vi "Main_FPGA_r1.vi"() -> ()   [LabVIEW 2018]
uses:
  <vilib>/rvi/Emulation/niFpgaGetClockAttributes.vi
  <vilib>/rvi/Emulation/niFpgaSctlEmulationGetInTimedLoop.vi
  <vilib>/rvi/Emulation/niFpgaEmulationReportErrorSimple.vi
  <vilib>/rvi/Emulation/niFpgaCriticalErrorInLSC.vi
  <vilib>/rvi/Emulation/niFpgaProcessEmulError.vi
  SubVI/24AIO/AO/AO_FPGA.lvlib
  SubVI/24AIO/AI/AI_FPGA.lvlib
panel:
  out "AI19-26[]":i16[](array[numeric])
  out "AI10-17[]":i16[](array[numeric])
  out "AI1-8[]":i16[](array[numeric])
  in  "InitializeAI?":bool caption="Initialize?"
  in  "AO_Data(U32)":u32
  # "AI"
  # "AO"
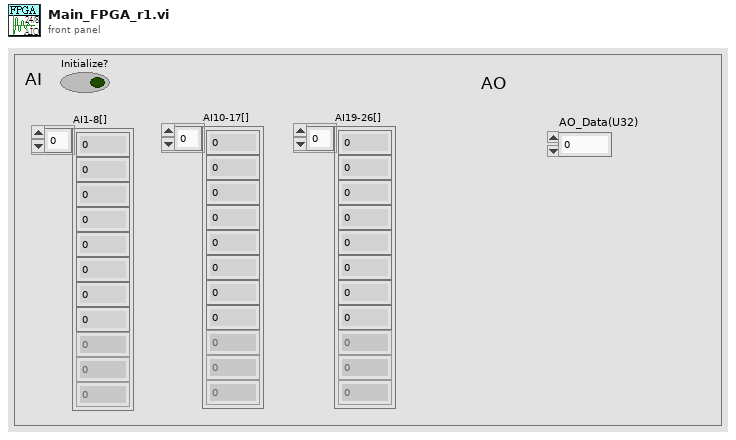
[diagram p1: front panel]
types:
  T1 = cluster{"CS":refnum<k21>, "CLK":refnum<k21>, "MOSI":refnum<k21>}
  T2 = cluster{"CONV":refnum<k21>, "RST":refnum<k21>, "SCK":refnum<k21>, "CS":refnum<k21>, "BUSY":refnum<k21>, "DOUT_A":refnum<k21>, "DOUT_B":refnum<k21>, "t_RST (ticks)":u32, "t_CONV (ticks)":u32, "t_BUSYMAX (ticks)":u32}
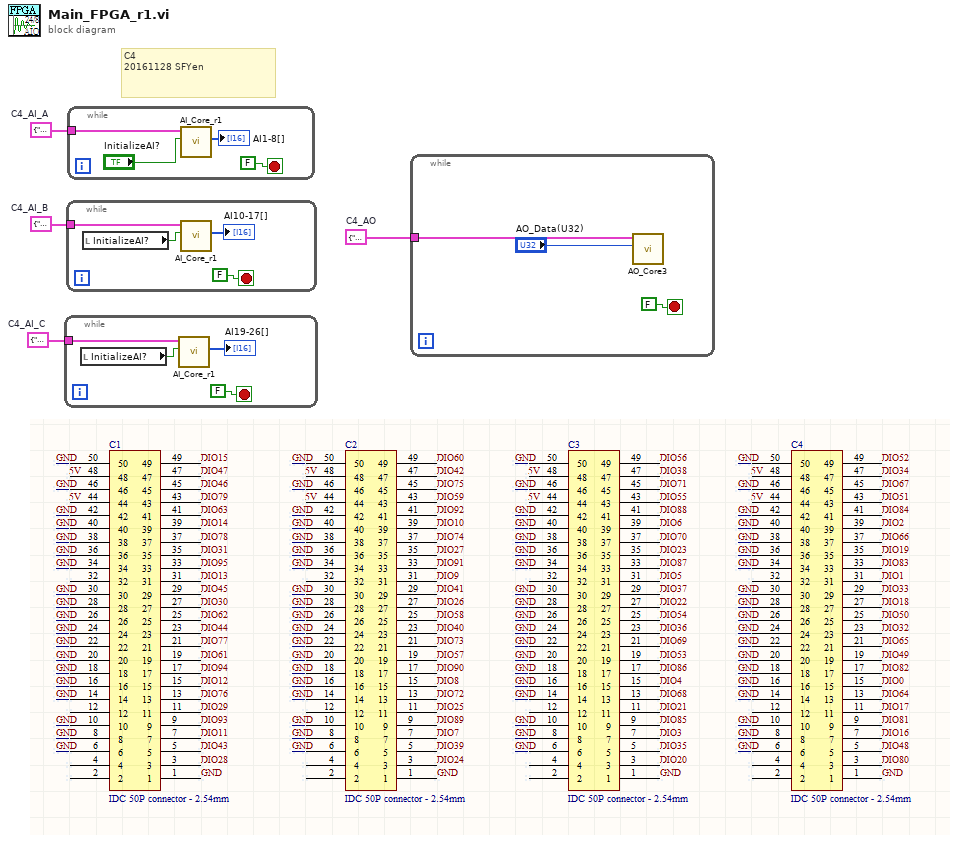
[diagram p0: block diagram]
diagram:
  w4 = T1 {"CS"="RMC/DIO67", "CLK"="RMC/DIO52", "MOSI"="RMC/DIO34"}  # C4_AO
  w1 = T2 {"CONV"="RMC/DIO51", "RST"="RMC/DIO84", "SCK"="RMC/DIO2", "CS"="RMC/DIO66", "BUSY"="RMC/DIO19", "DOUT_A"="RMC/DIO83", "DOUT_B"="RMC/DIO1", "t_RST (ticks)"=0, "t_CONV (ticks)"=0, "t_BUSYMAX (ticks)"=0}  # C4_AI_C
  w2 = T2 {"CONV"="RMC/DIO33", "RST"="RMC/DIO18", "SCK"="RMC/DIO50", "CS"="RMC/DIO32", "BUSY"="RMC/DIO65", "DOUT_A"="RMC/DIO49", "DOUT_B"="RMC/DIO82", "t_RST (ticks)"=0, "t_CONV (ticks)"=0, "t_BUSYMAX (ticks)"=0}  # C4_AI_B
  w3 = T2 {"CONV"="RMC/DIO0", "RST"="RMC/DIO64", "SCK"="RMC/DIO17", "CS"="RMC/DIO81", "BUSY"="RMC/DIO16", "DOUT_A"="RMC/DIO48", "DOUT_B"="RMC/DIO80", "t_RST (ticks)"=0, "t_CONV (ticks)"=0, "t_BUSYMAX (ticks)"=0}  # C4_AI_A
  # "C4\n20161128 SFYen"
  n1 = while {
    tunnel: w1 -> [w8]
    stop <- FALSE stop-if-true
    n2 = local read "InitializeAI?"() -> (w6:bool)
    n3 = call "AI_Core_r1.vi"("InitializeAI?"=w6, "AI_Pin_Cluster"=w8) -> ("8Ch_Data[]"=→"AI19-26[]":i16[])  [unwired: 9 in]
  }
  n4 = while {
    tunnel: w2 -> [w12]
    stop <- FALSE stop-if-true
    n5 = local read "InitializeAI?"() -> (w10:bool)
    n6 = call "AI_Core_r1.vi"("InitializeAI?"=w10, "AI_Pin_Cluster"=w12) -> ("8Ch_Data[]"=→"AI10-17[]":i16[])  [unwired: 9 in]
  }
  n7 = while {
    tunnel: w3 -> [w16]
    stop <- FALSE stop-if-true
    n8 = call "AI_Core_r1.vi"("InitializeAI?"="InitializeAI?", "AI_Pin_Cluster"=w16) -> ("8Ch_Data[]"=→"AI1-8[]":i16[])  [unwired: 9 in]
  }
  n9 = while {
    tunnel: w4 -> [w18]
    stop <- FALSE stop-if-true
    n10 = call "AO_Core3.vi"("data"="AO_Data(U32)", "Spi_A"=w18) -> ()  [unwired: 9 in, 1 out]
  }
